vi "DSF.Engine.Hardware Info.Get CPU.vi"(8 "error in (no error)":errorcluster, 11 "Hardware Info in":refnum<class "DSF.Engine.Hardware Info.lvclass">) -> (0 "error out":errorcluster, 2 "CPU Info":refnum<class "DSF.Engine.Hardware Info.CPU.lvclass">, 3 "Hardware Info out":refnum<class "DSF.Engine.Hardware Info.lvclass">)   [LabVIEW 2017, in "Data Sharing Framework Engine.lvlib" / "DSF.Engine.Hardware Info.lvclass"]
uses:
  DSF.Engine.Hardware Info.lvclass
  DSF.Engine.Hardware Info.CPU.lvclass
  DSF.Engine.Hardware Info.lvclass/DSF.Engine.Hardware Info.ctl
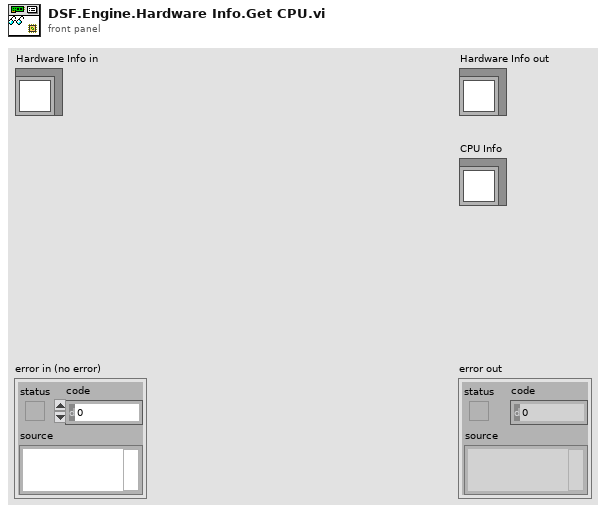
[diagram p1: front panel]
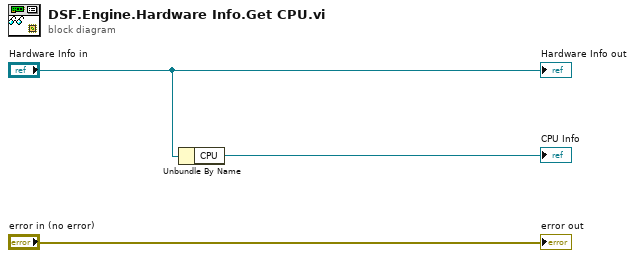
[diagram p0: block diagram]
diagram:
  n1 = Unbundle By Name("Hardware Info in") -> ("CPU"=→"CPU Info":refnum<class "DSF.Engine.Hardware Info.CPU.lvclass">)
  "error out" <- "error in (no error)"
  "Hardware Info out" <- "Hardware Info in"
